vi "Delete TTL.vi"(8 "error in (no error)":errorcluster, 10 "Name":string, 11 "State in":refnum<class "State.lvclass">) -> (0 "error out":errorcluster, 3 "State out":refnum<class "State.lvclass">)   [LabVIEW 2015, in "State.lvclass"]
uses:
  State.lvclass
  State.lvclass/State.ctl
  Termination/Termination.lvclass/Termination.ctl
  TTL VIs/Control Classes/Base Class/TTLController.lvclass/TTLController.ctl
  Timeout/Timeout.lvclass/Timeout.ctl
  TTL VIs/Control Classes/Base Class/Read Name.vi
  Termination/Read TTL.vi
  Termination/Write TTL.vi
  Timeout/Read TTL.vi
  Timeout/Write TTL.vi
  TTL VIs/Control Classes/Base Class/TTLController.lvclass
  Timeout/Timeout.lvclass
  Termination/Termination.lvclass
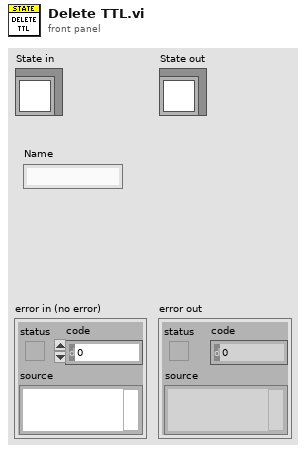
[diagram p1: front panel]
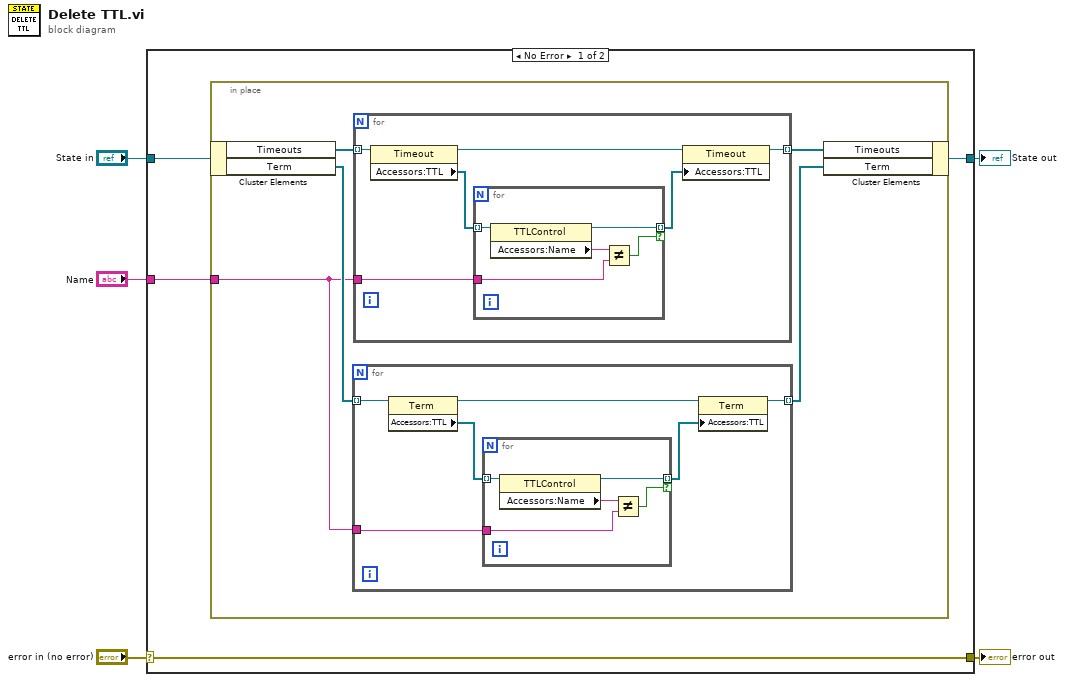
[diagram p0: block diagram]
diagram:
  n1 = case shown="No Error" "error in (no error)" {
    selector: "error in (no error)" -> [w9 w38]
    tunnel: [w9 w38] -> w4
    tunnel: [w7 w37] -> w2
    tunnel: "State in" -> [w8 w37]
    tunnel: "Name" -> [w6 _]
    frame No Error {
      n2 = in-place {
        in-place-border: w6 -> [w12]
        n3 = in-place-cluster #1(w8) -> ("Timeouts"=w14:refnum<class "Timeout.lvclass">[], "Term"=w13:refnum<class "Termination.lvclass">[])
        n4 = for {
          tunnel: w13 -> [w28] mode=indexing
          tunnel: w12 -> [w26]
          tunnel: [w27] -> w10 mode=indexing
          n5 = property class="Term"(reference=w28) -> (reference out=w30:refnum<class "Termination.lvclass">, "Accessors:TTL"=w31:refnum<class "TTLController.lvclass">[])  [unwired: 1 in, 1 out]
          n6 = for {
            tunnel: w31 -> [w36] mode=indexing
            tunnel: w26 -> [w34]
            tunnel: [w33] -> w29 mode=indexing if=w32
            n7 = property class="TTLControl"(reference=w36) -> (reference out=w33:refnum<class "TTLController.lvclass">, "Accessors:Name"=w35:string)  [unwired: 1 in, 1 out]
            n8 = Not Equal?(x=w35, y=w34) -> (x != y?=w32:bool)
          }
          n9 = property class="Term"(reference=w30, "Accessors:TTL"=w29) -> (reference out=w27:refnum<class "Termination.lvclass">)  [unwired: 1 in, 1 out]
        }
        n10 = for {
          tunnel: w14 -> [w19] mode=indexing
          tunnel: w12 -> [w18]
          tunnel: [w15] -> w11 mode=indexing
          n11 = property class="Timeout"(reference=w19) -> (reference out=w17:refnum<class "Timeout.lvclass">, "Accessors:TTL"=w20:refnum<class "TTLController.lvclass">[])  [unwired: 1 in, 1 out]
          n12 = for {
            tunnel: w20 -> [w25] mode=indexing
            tunnel: w18 -> [w23]
            tunnel: [w22] -> w16 mode=indexing if=w21
            n13 = property class="TTLControl"(reference=w25) -> (reference out=w22:refnum<class "TTLController.lvclass">, "Accessors:Name"=w24:string)  [unwired: 1 in, 1 out]
            n14 = Not Equal?(x=w24, y=w23) -> (x != y?=w21:bool)
          }
          n15 = property class="Timeout"(reference=w17, "Accessors:TTL"=w16) -> (reference out=w15:refnum<class "Timeout.lvclass">)  [unwired: 1 in, 1 out]
        }
        n16 = in-place-cluster #1("Timeouts"=w11, "Term"=w10) -> (w7:refnum<class "State.lvclass">)
      }
    }
    frame Error {
    }
  }
  "error out" <- w4
  "State out" <- w2
